vi "updateDest.vi"(8 "error in (no error)":errorcluster, 10 "NewAllyRobots":refnum<class "Robot.lvclass">[](array[class]), 11 "LastAlly":refnum<class "Ally.lvclass">) -> (0 "error out":errorcluster, 2 "NewAllyRobotsUpdated":refnum<class "Robot.lvclass">[](array[class]), 3 "Ally out":refnum<class "Ally.lvclass">)   [LabVIEW 2023, in "Ally.lvclass"]
uses:
  Ally.lvclass
  Robot_class/Robot.lvclass
  Utilities_class/Utilities.lvclass
  Team_class/Team.lvclass/Team.ctl
  Robot_class/Robot.lvclass/Robot.ctl
  Robot_class/Write dest_x.vi
  Robot_class/Write dest_y.vi
  Robot_class/Write dest_orientation.vi
  Robot_class/Write dest_x_kick.vi
  Robot_class/Write dest_y_kick.vi
  Robot_class/Write tactic.vi
  Robot_class/Read id.vi
  Robot_class/Read dest_x.vi
  Robot_class/Read dest_y.vi
  Robot_class/Read dest_orientation.vi
  Robot_class/Read dest_x_kick.vi
  Robot_class/Read dest_y_kick.vi
  Robot_class/Read tactic.vi
  Team_class/Read RobotRef.vi
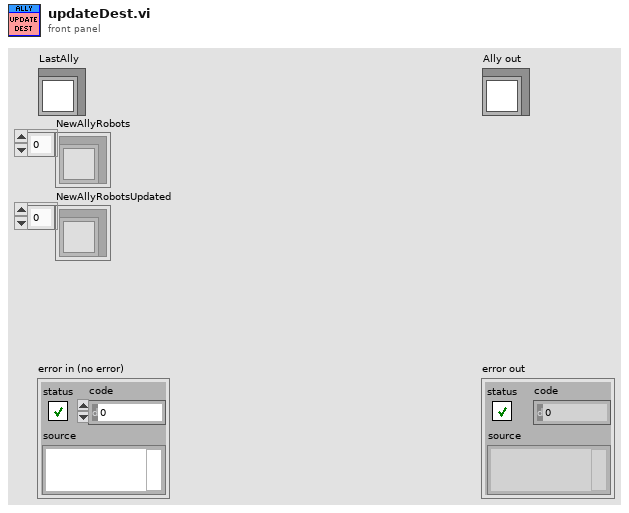
[diagram p1: front panel]
types:
  T1 = typedef "tactics.ctl" = enum16{"ReceivePassInFuturePoint", "Roller", "PrepareRollToPassRollerGoTo", "PrepareRollToPassReceiverGoTo", "WaitRoll", "PositionToRoll", "PenaltyAttacker", "PassObserver", "PenaltyDefense", "TableReceiverTactic", "Test", "DefendGoal", "Marker", "FollowAttacker", "DefendArea", "Shoot", "AttackerAimGoal", "AttackerBallOutOfField", "AttackerBlock", "AttackerStop", "Duelist", "Halt", "ZigZag", "GoTo", "Timeout", "KickToPassReceiver", "PositionToReceivePass", "DefendAreaVSS", "DefendGoalVSS", "KickVSS", "AttackVSS", "DispBallVSS", "PenaltyAttackVSS", "WaitPass"}
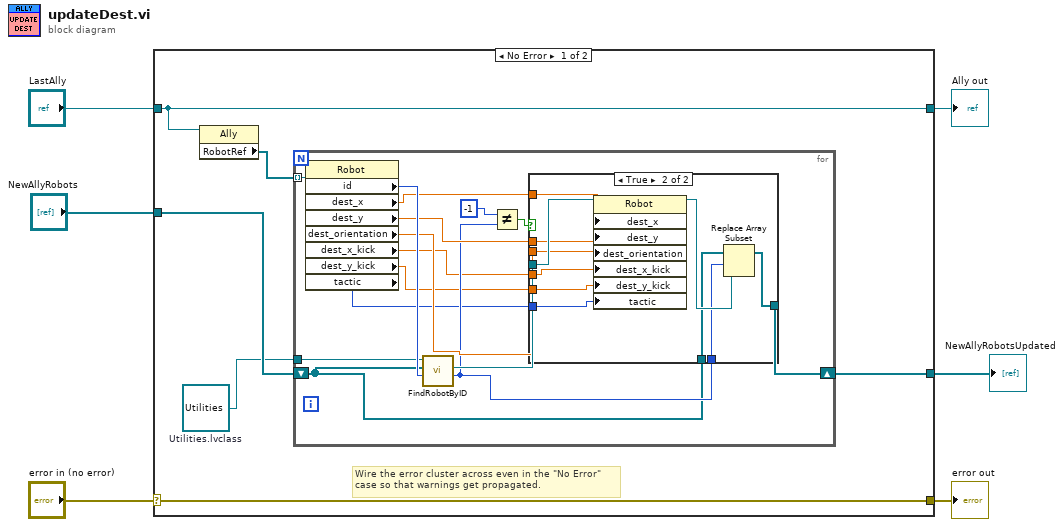
[diagram p0: block diagram]
diagram:
  n1 = case shown="No Error" "error in (no error)" {
    selector: "error in (no error)" -> [w12 w41]
    tunnel: [w12 w41] -> w5
    tunnel: [w11 w40] -> w3
    tunnel: "LastAlly" -> [w11 w40]
    tunnel: "NewAllyRobots" -> [w10 _]
    tunnel: [w7 _] -> w1
    frame No Error {
      w8 = refnum<class "Utilities.lvclass"> refnum  # Utilities.lvclass
      # "Wire the error cluster across even in the \"No Error\"\ncase so that warnings get propagated."
      n2 = property class="Ally"(reference=w11) -> ("RobotRef"=w9:refnum<class "Robot.lvclass">[])  [unwired: 1 in, 2 out]
      n3 = for {
        tunnel: w9 -> [w27] mode=indexing
        tunnel: w8 -> [w19]
        shift-right: [w16] -> w7
        shift-left: w10 -> [w17]
        n4 = property class="Robot"(reference=w27) -> ("id"=w26:i32, "dest_x"=w23:dbl, "dest_y"=w22:dbl, "dest_orientation"=w21:dbl, "dest_x_kick"=w15:dbl, "dest_y_kick"=w14:dbl, "tactic"=w13:T1)  [unwired: 1 in, 2 out]
        n5 = call-dynamic "FindRobotByID.vi"("id"=w26, "RobotRef"=w17, "Utilities in"=w19) -> ("index"=w18:i32, "Robot"=w24:refnum<class "Robot.lvclass">)  [unwired: 5 in, 2 out]
        n6 = Not Equal?(x=-1 ("y"), y=w18) -> (x != y?=w20:bool)
        n7 = case shown="True" w20 {
          tunnel: w24 -> [_ w39]
          tunnel: w23 -> [_ w38]
          tunnel: w22 -> [_ w37]
          tunnel: w21 -> [_ w36]
          tunnel: w18 -> [_ w34]
          tunnel: w17 -> [w28 w33]
          tunnel: [w28 w32] -> w16
          tunnel: w15 -> [_ w31]
          tunnel: w14 -> [_ w30]
          tunnel: w13 -> [_ w29]
          frame False {
          }
          frame True {
            n8 = property class="Robot"(reference=w39, "dest_x"=w38, "dest_y"=w37, "dest_orientation"=w36, "dest_x_kick"=w31, "dest_y_kick"=w30, "tactic"=w29) -> (reference out=w35:refnum<class "Robot.lvclass">)  [unwired: 1 in, 1 out]
            n9 = Replace Array Subset(array=w33, new element=w35, index=w34) -> (w32:refnum<class "Robot.lvclass">[])
          }
        }
      }
    }
    frame Error {
    }
  }
  "error out" <- w5
  "Ally out" <- w3
  "NewAllyRobotsUpdated" <- w1
